vi "Unregister by Name.vi"(7 "Event":refnum<class "Event.lvclass">, 8 "error in (no error)":errorcluster, 10 "View Name":string, 11 "Controller in":refnum<class "Controller.lvclass">) -> (0 "error out":errorcluster, 3 "Controller out":refnum<class "Controller.lvclass">)   [LabVIEW 2023, in "MVC Actors.lvlib" / "Controller.lvclass"]
doc: "Lets a View specified by <b>View Name</b> register an <b>Event</b> to the Controller."
uses:
  Controller.lvclass
  Event/Event.lvclass
  Controller.lvclass/Controller.ctl
  View Details.ctl
  <vilib>/ActorFramework/Message Enqueuer/Message Enqueuer.lvclass
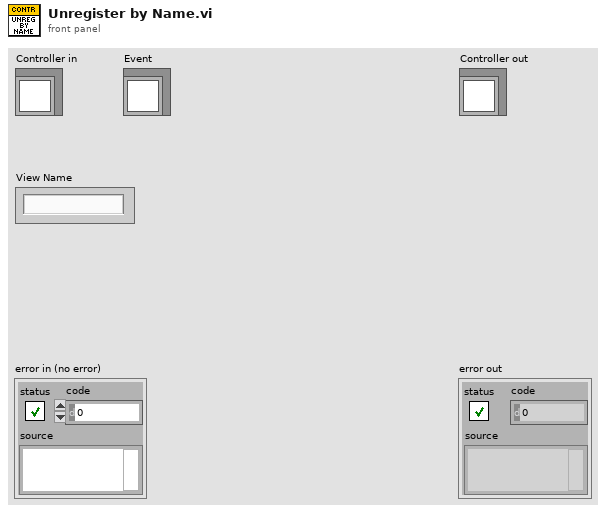
[diagram p1: front panel]
types:
  T1 = typedef "MVC Actors.lvlib/Controller.lvclass/View Details.ctl" = cluster{"Exclude From Broadcast":bool, "Receive Only":bool, "Paused":bool, "View Enqueuer":refnum<class "Message Enqueuer.lvclass">}
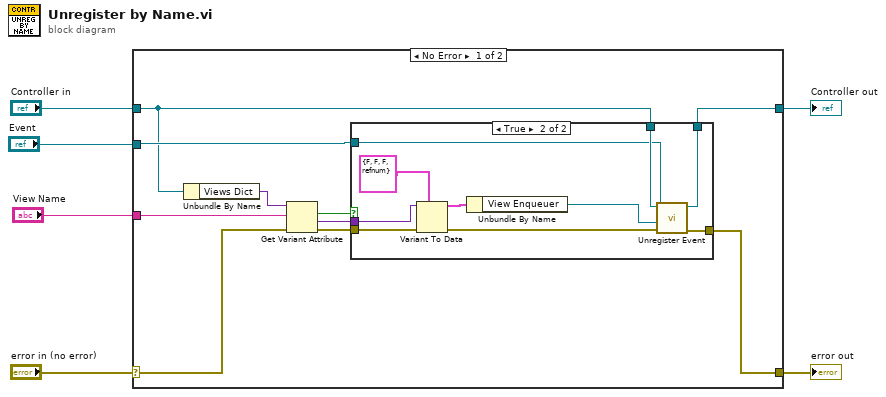
[diagram p0: block diagram]
diagram:
  n1 = case shown="No Error" "error in (no error)" {
    selector: "error in (no error)" -> [w8 w30]
    tunnel: [w7 w30] -> w5
    tunnel: [w9 w29] -> w3
    tunnel: "Controller in" -> [w10 w29]
    tunnel: "View Name" -> [w15 _]
    tunnel: "Event" -> [w11 _]
    frame No Error {
      n2 = Unbundle By Name(w10) -> ("Views Dict"=w16:variant)
      n3 = Get Variant Attribute(Variant=w16, name=w15, error in=w8) -> (found=w14:bool, value=w13:variant, error out=w12:errorcluster)  [unwired: 1 in, 1 out]
      n4 = case shown="True" w14 {
        tunnel: w13 -> [_ w27]
        tunnel: w12 -> [w18 w28]
        tunnel: w10 -> [w17 w24]
        tunnel: w11 -> [_ w23]
        tunnel: [w18 w22] -> w7
        tunnel: [w17 w21] -> w9
        frame False {
        }
        frame True {
          n5 = Variant To Data(error in=w28, type=T1 {"Exclude From Broadcast"=FALSE, "Receive Only"=FALSE, "Paused"=FALSE, "View Enqueuer"=refnum} ("Message Enqueuer"), Variant=w27) -> (data=w25:T1, error out=w26:errorcluster)
          n6 = Unbundle By Name(w25) -> ("View Enqueuer"=w19:refnum<class "Message Enqueuer.lvclass">)
          n7 = call "Unregister Event.vi"("Error In"=w26, "Registrant Address"=w19, "Event"=w23, "Controller Actor In"=w24) -> ("Error Out"=w22:errorcluster, "Controller Actor Out"=w21:refnum<class "Controller.lvclass">)  [unwired: 6 in]
        }
      }
    }
    frame Error {
    }
  }
  "error out" <- w5
  "Controller out" <- w3
